vi "getCounterPosition.vi"(0 "MultiAxisController in":refnum<class "_MultiAxisController.lvclass">, 2 "type (def = ENCODER)":T2, 5 "error in (no error)":errorcluster) -> (14 "MultiAxisController out":refnum<class "_MultiAxisController.lvclass">, 16 "counter_vals (out)":T1, 19 "error out":errorcluster)   [LabVIEW 2020, in "classes.lvlib" / "_MultiAxisController.lvclass"]
doc: "Get the encoder counter position\n\nProduced By:\n\n<B>Kod Integrations, LLC</B>\n4835 Marianne Drive\nMount Airy, MD 21771\nhttp://www.kodintegrations.com\nemail: info@kodintegrations.com\nphone: (240) 687-1288"
uses:
  _MultiAxisController.lvclass
  C:/GEECS/Developers Version/source/Device Drivers/Newmark-NSC-A/Arcus Driver 3.0.0/ArcusUsbComm/classes/Controller/_Controller.lvclass
  common/controls/counter_type.ctl
  common/controls/counter_values.ctl
  Controller/_Controller.lvclass
  libraries/common.lvlib
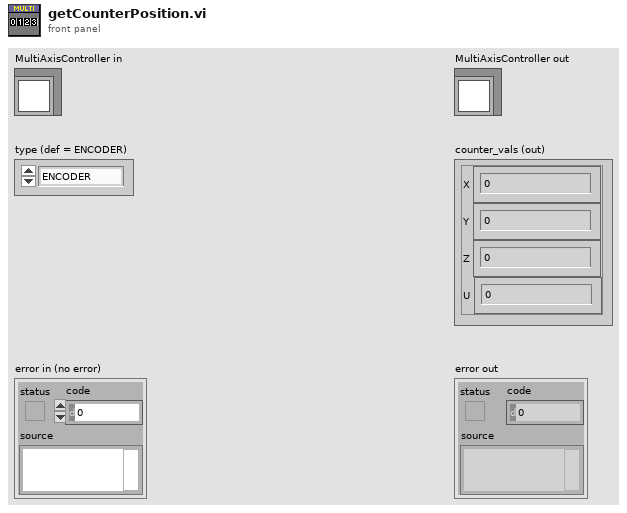
[diagram p1: front panel]
types:
  T1 = typedef "common.lvlib/counter_values.ctl" = cluster{"X":i32, "Y":i32, "Z":i32, "U":i32}
  T2 = typedef "common.lvlib/counter_type.ctl" = enum16{"ENCODER", "PULSE"}
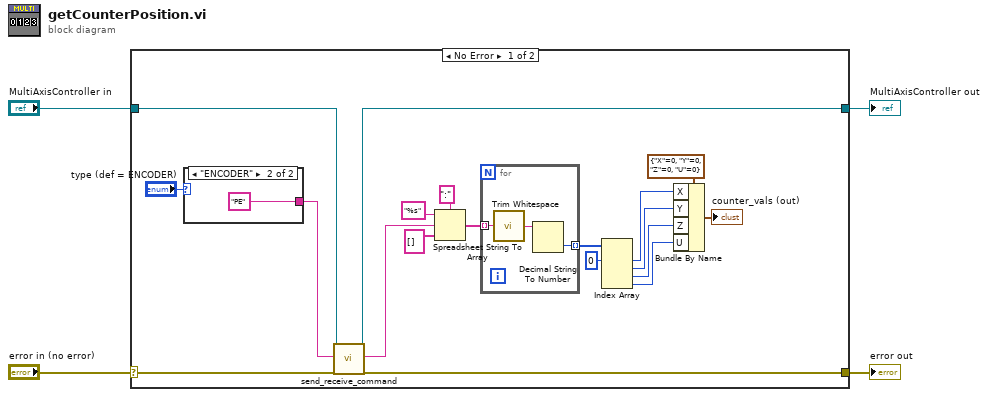
[diagram p0: block diagram]
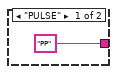
[diagram p2: hidden frame]
diagram:
  n1 = case shown="No Error" "error in (no error)" {
    selector: "error in (no error)" -> [w22 w30]
    tunnel: [w21 w30] -> w3
    tunnel: [w18 w29] -> w1
    tunnel: "MultiAxisController in" -> [w19 w29]
    frame No Error {
      n2 = case shown="\"ENCODER\"" "type (def = ENCODER)" {
        tunnel: ["PP" "PE"] -> w20
        frame "PULSE" {
        }
        frame "ENCODER" {
        }
      }
      n3 = call "send_receive_command.vi"("reference (in)"=w19, "ASCII Command (in)"=w20, "error in (no error)"=w22) -> ("reference (out)"=w18:refnum<class "_MultiAxisController.lvclass">, "response (out)"=w16:string, "error out"=w21:errorcluster)  [unwired: 12 in, 2 out]
      n4 = Spreadsheet String To Array(delimiter (Tab)=":", format string="%s", spreadsheet string=w16, array type (2D Dbl)=string[] []) -> (array=w13:string[])
      n5 = for {
        tunnel: w13 -> [w26] mode=indexing
        tunnel: [w24] -> w12 mode=indexing
        n6 = call <vilib>:"Trim Whitespace.vi"("string"=w26) -> ("trimmed string"=w25:string)  [unwired: 1 in]
        n7 = Decimal String To Number(string=w25) -> (number=w24:i32)  [unwired: 2 in, 1 out]
      }
      n8 = Index Array(array=w12, index #1=0 ("index")) -> (element #1=w9:i32, element #2=w8:i32, element #3=w7:i32, element #4=w6:i32)  [unwired: 3 in]
      n9 = Bundle By Name(cluster=T1 {"X"=0, "Y"=0, "Z"=0, "U"=0} ("counter_vals (out)"), "X"=w9, "Y"=w8, "Z"=w7, "U"=w6) -> (→"counter_vals (out)":T1)
    }
    frame Error {
    }
  }
  "error out" <- w3
  "MultiAxisController out" <- w1
